vi "niSYS - SG - GEN - UTIL - Apply Headroom.vi"(0 "Complex Signal In":cluster{"x0":dbl, "dx":dbl, "y":cdb[]} {"y" format="%.2f"; "dx" format="%^.2e"; "x0" format="%^.2e"}, 5 "Headroom, dB (-1 = Auto)":dbl=-1.0 format="%.1f", 11 "error in (no error)":errorcluster) -> (4 "Complex Signal Out":cluster{"x0":dbl, "dx":dbl, "y":cdb[]} {"y" format="%.2f"; "dx" format="%^.2e"; "x0" format="%^.2e"}, 6 "Actual Headroom, dB":dbl format="%.1f", 15 "error out":errorcluster)   [LabVIEW 2020]
doc: "(c) Copyright 2006, National Instruments, Inc. This VI may not be duplicated, sold, or distributed without written consent from National Instruments."
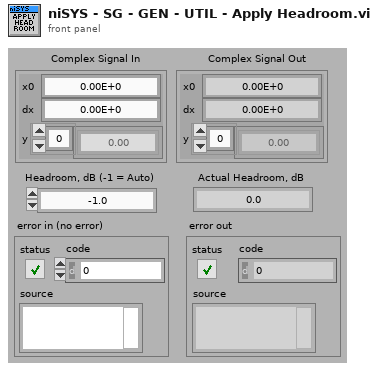
[diagram p1: front panel]
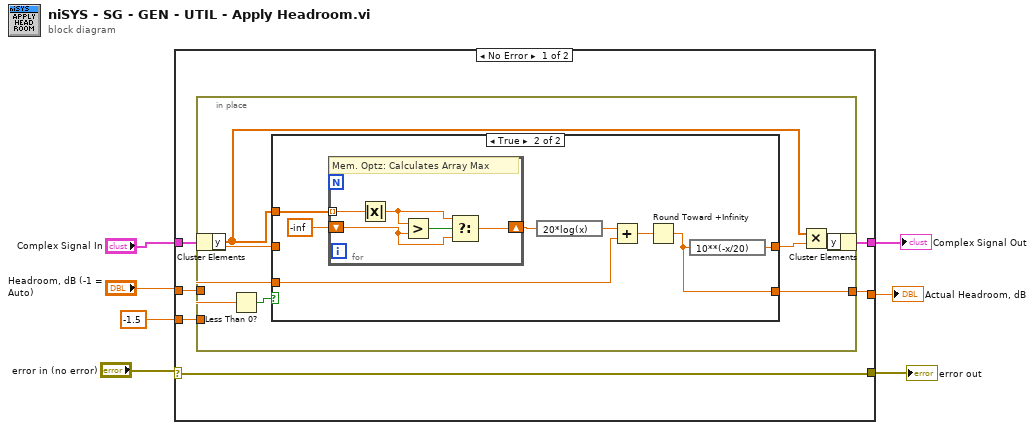
[diagram p0: block diagram]
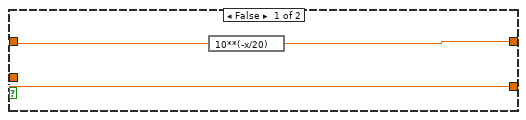
[diagram p2: hidden frame]
diagram:
  n1 = case shown="No Error" "error in (no error)" {
    selector: "error in (no error)" -> [w12 w38]
    tunnel: "Complex Signal In" -> [w10 w37]
    tunnel: [w12 w38] -> w7
    tunnel: "Headroom, dB (-1 = Auto)" -> [w13 w36]
    tunnel: [w9 w37] -> w4
    tunnel: [w11 w36] -> w3
    tunnel: -1.5 -> [w8 _]
    frame No Error {
      n2 = in-place {
        in-place-border: w13 -> [w14]
        in-place-border: [w19] -> w11
        in-place-border: w8 -> [w16]
        n3 = in-place-cluster #1(w10) -> ("y"=w18:cdb[])
        n4 = Less Than 0?(x=w14) -> (x < 0?=w15:bool)
        n5 = case shown="True" w15 {
          tunnel: [w22 w29] -> w20
          tunnel: w14 -> [w21 _]
          tunnel: w18 -> [_ w25]
          tunnel: [w21 w30] -> w19
          tunnel: w16 -> [_ w27]
          frame False {
            n6 = expression code="10**(-x/20)"(w21) -> (w22:dbl)
          }
          frame True {
            n7 = for {
              tunnel: w25 -> [w35] mode=indexing
              shift-right: [w31] -> w24
              shift-left: -inf -> [w32]
              # "Mem. Optz: Calculates Array Max"
              n8 = Absolute Value(x=w35) -> (abs(x)=w33:dbl)
              n9 = Greater?(x=w33, y=w32) -> (0:w34:bool)
              n10 = Select(t=w33, s=w34, f=w32) -> (s? t:f=w31:dbl)
            }
            n11 = expression code="20*log(x)"(w24) -> (w28:dbl)
            n12 = Add(x=w28, y=w27) -> (x+y=w26:dbl)
            n13 = Round Toward +Infinity(x=w26) -> (ceil(x): smallest int >= x=w30:dbl)
            n14 = expression code="10**(-x/20)"(w30) -> (w29:dbl)
          }
        }
        n15 = Multiply(x=w18, y=w20) -> (x*y=w17:cdb[])
        n16 = in-place-cluster #1("y"=w17) -> (w9:cluster{"x0":dbl, "dx":dbl, "y":cdb[]})
      }
    }
    frame Error {
    }
  }
  "error out" <- w7
  "Complex Signal Out" <- w4
  "Actual Headroom, dB" <- w3
